vi "Format_ZCAN_TransmitFD_Data.vi"(6 "fd_additional _flags":u32, 7 "Agreement":T1=enum."CANFD", 8 "Send_string_data":string, 9 "frame_format":i16, 10 "frame_type":i16, 11 "can_frame.can_id":u32) -> (3 "tagZCAN_TransmitFD_Data":T2)   [LabVIEW 2020, in "zlgcan.lvlib"]
uses:
  zlgcan.lvlib
  data_type/tagZCAN_TransmitFD_Data.ctl
  data_type/canfd_frame.ctl
  data_type/Agreement.ctl
panel:
  # "s"
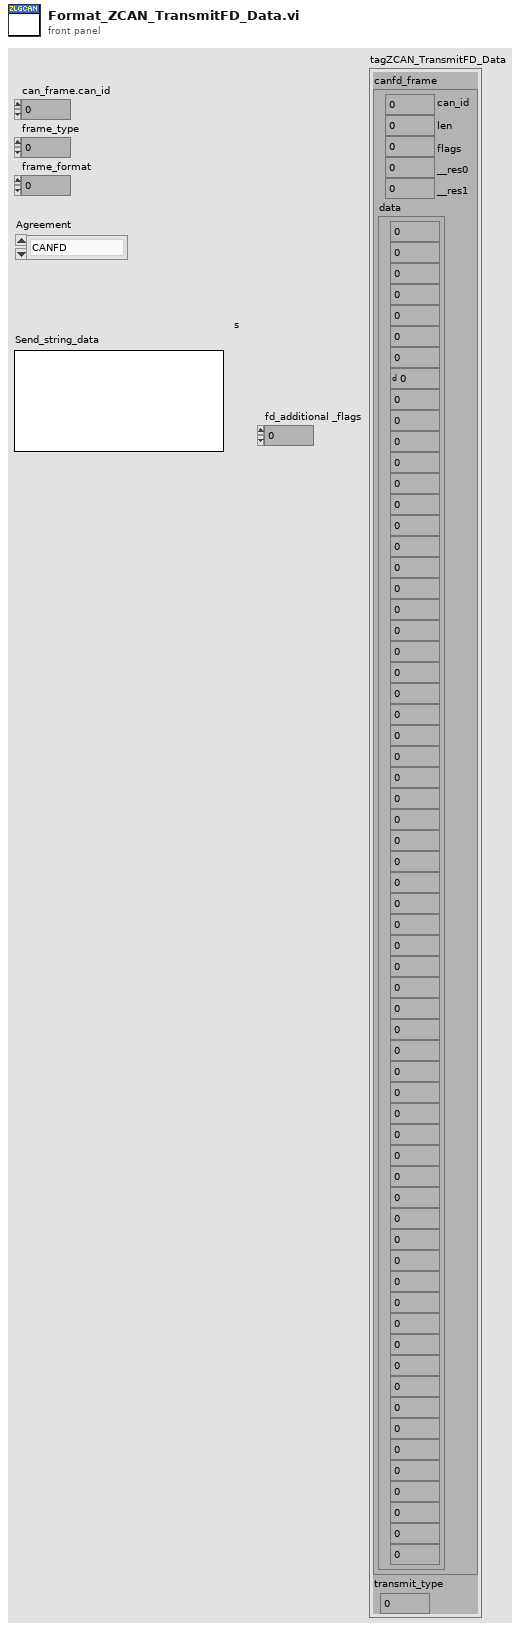
[diagram p1: front panel]
types:
  T1 = typedef "zlgcan.lvlib/Agreement.ctl" = enum16{"CAN", "CANFD"}
  T2 = typedef "zlgcan.lvlib/tagZCAN_TransmitFD_Data.ctl" = cluster{"canfd_frame":T3, "transmit_type":u32}
  T3 = typedef "zlgcan.lvlib/canfd_frame.ctl" = cluster{"can_id":u32, "len":u8, "flags":u8, "__res0":u8, "__res1":u8, "data":cluster{"CAN数据[0]":u8, "CAN数据[1]":u8, "CAN数据[2]":u8, "CAN数据[3]":u8, "CAN数据[4]":u8, "CAN数据[5]":u8, "CAN数据[6]":u8, "CAN数据[7]":u8, "CAN数据[8]":u8, "CAN数据[9]":u8, "CAN数据[10]":u8, "CAN数据[11] ":u8, "CAN数据[12] ":u8, "CAN数据[13] ":u8, "CAN数据[14] ":u8, "CAN数据[15] ":u8, "CAN数据[16]":u8, "CAN数据[17]":u8, "CAN数据[18]":u8, "CAN数据[19]":u8, "CAN数据[20]":u8, "CAN数据[21]":u8, "CAN数据[22]":u8, "CAN数据[23]":u8, "CAN数据[24] ":u8, "CAN数据[25]":u8, "CAN数据[26]":u8, "CAN数据[27]":u8, "CAN数据[28]":u8, "CAN数据[29]":u8, "CAN数据[30]":u8, "CAN数据[31]":u8, "CAN数据[32]":u8, "CAN数据[33]":u8, "CAN数据[34]":u8, "CAN数据[35]":u8, "CAN数据[36]":u8, "CAN数据[37]":u8, "CAN数据[38]":u8, "CAN数据[39]":u8, "CAN数据[40]":u8, "CAN数据[41]":u8, "CAN数据[42]":u8, "CAN数据[43]":u8, "CAN数据[44]":u8, "CAN数据[45]":u8, "CAN数据[46]":u8, "CAN数据[47]":u8, "CAN数据[48]":u8, "CAN数据[49]":u8, "CAN数据[50]":u8, "CAN数据[51]":u8, "CAN数据[52]":u8, "CAN数据[53]":u8, "CAN数据[54]":u8, "CAN数据[55]":u8, "CAN数据[56]":u8, "CAN数据[57]":u8, "CAN数据[58]":u8, "CAN数据[59]":u8, "CAN数据[60]":u8, "CAN数据[61]":u8, "CAN数据[62]":u8, "CAN数据[63]":u8}}
  T4 = cluster{"[0]":u32, "[1]":u32, "[2]":u32, "[3]":u32, "[4]":u32, "[5]":u32, "[6]":u32, "[7]":u32, "[8]":u32, "[9]":u32, "[10]":u32, "[11]":u32, "[12]":u32, "[13]":u32, "[14]":u32, "[15]":u32, "[16]":u32, "[17]":u32, "[18]":u32, "[19]":u32, "[20]":u32, "[21]":u32, "[22]":u32, "[23]":u32, "[24]":u32, "[25]":u32, "[26]":u32, "[27]":u32, "[28]":u32, "[29]":u32, "[30]":u32, "[31]":u32, "[32]":u32, "[33]":u32, "[34]":u32, "[35]":u32, "[36]":u32, "[37]":u32, "[38]":u32, "[39]":u32, "[40]":u32, "[41]":u32, "[42]":u32, "[43]":u32, "[44]":u32, "[45]":u32, "[46]":u32, "[47]":u32, "[48]":u32, "[49]":u32, "[50]":u32, "[51]":u32, "[52]":u32, "[53]":u32, "[54]":u32, "[55]":u32, "[56]":u32, "[57]":u32, "[58]":u32, "[59]":u32, "[60]":u32, "[61]":u32, "[62]":u32, "[63]":u32}
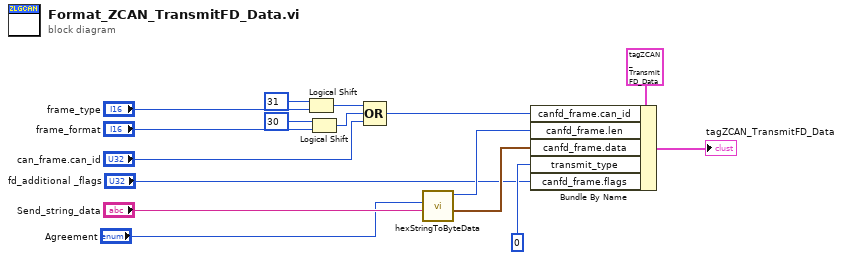
[diagram p0: block diagram]
diagram:
  n1 = Logical Shift(y=i16 31, x="frame_type") -> (x << y=w15:i16)
  n2 = Logical Shift(y=i16 30, x="frame_format") -> (x << y=w12:i16)
  n3 = Compound Arithmetic op=OR ("复合运算")(w15, w12, "can_frame.can_id") -> (w11:u32)
  n4 = call "hexStringToByteData.vi"("数据输入"="Send_string_data", "协议"="Agreement") -> ("CANFD_data"=w3:T4, "字节数"=w9:u8)  [unwired: 6 in, 2 out]
  n5 = Bundle By Name(cluster=T2 {"canfd_frame"={"can_id"=0, "len"=0, "flags"=0, "__res0"=0, "__res1"=0, "data"={"CAN数据[0]"=0, "CAN数据[1]"=0, "CAN数据[2]"=0, "CAN数据[3]"=0, "CAN数据[4]"=0, "CAN数据[5]"=0, "CAN数据[6]"=0, "CAN数据[7]"=0, "CAN数据[8]"=0, "CAN数据[9]"=0, "CAN数据[10]"=0, "CAN数据[11] "=0, "CAN数据[12] "=0, "CAN数据[13] "=0, "CAN数据[14] "=0, "CAN数据[15] "=0, "CAN数据[16]"=0, "CAN数据[17]"=0, "CAN数据[18]"=0, "CAN数据[19]"=0, "CAN数据[20]"=0, "CAN数据[21]"=0, "CAN数据[22]"=0, "CAN数据[23]"=0, "CAN数据[24] "=0, "CAN数据[25]"=0, "CAN数据[26]"=0, "CAN数据[27]"=0, "CAN数据[28]"=0, "CAN数据[29]"=0, "CAN数据[30]"=0, "CAN数据[31]"=0, "CAN数据[32]"=0, "CAN数据[33]"=0, "CAN数据[34]"=0, "CAN数据[35]"=0, "CAN数据[36]"=0, "CAN数据[37]"=0, "CAN数据[38]"=0, "CAN数据[39]"=0, "CAN数据[40]"=0, "CAN数据[41]"=0, "CAN数据[42]"=0, "CAN数据[43]"=0, "CAN数据[44]"=0, "CAN数据[45]"=0, "CAN数据[46]"=0, "CAN数据[47]"=0, "CAN数据[48]"=0, "CAN数据[49]"=0, "CAN数据[50]"=0, "CAN数据[51]"=0, "CAN数据[52]"=0, "CAN数据[53]"=0, "CAN数据[54]"=0, "CAN数据[55]"=0, "CAN数据[56]"=0, "CAN数据[57]"=0, "CAN数据[58]"=0, "CAN数据[59]"=0, "CAN数据[60]"=0, "CAN数据[61]"=0, "CAN数据[62]"=0, "CAN数据[63]"=0}}, "transmit_type"=0} ("tagZCAN_TransmitFD_Data 2"), "canfd_frame.can_id"=w11, "canfd_frame.len"=w9, "canfd_frame.data"=w3, "transmit_type"=u32 0, "canfd_frame.flags"="fd_additional _flags") -> (→"tagZCAN_TransmitFD_Data":T2)
